vi "Demo_3 - Channel device_SetXYZRange.vi"() -> ()   [LabVIEW 2011]
uses:
  <instrlib>/Thorlabs_MDT69xB/Thorlabs_MDT69xB.lvlib
panel:
  out "Get Z voltage(V)":dbl
  out "Get Y voltage(V)":dbl
  out "Get X voltage(V)":dbl
  in  "Set Z Voltage(V)":dbl
  in  "Set Y Voltage(V)":dbl
  in  "Set x Voltage(V)":dbl
  out "Get z max voltage(V)":dbl
  out "Get z min voltage(V)":dbl
  out "Get y max voltage(V)":dbl
  out "Get y min voltage(V)":dbl
  in  "Set z max Voltage(V)":dbl=75.0
  in  "Set z min Voltage(V)":dbl
  in  "Set y max Voltage(V)":dbl=75.0
  in  "Set y min Voltage(V)":dbl
  out "Get x max voltage(V)":dbl
  out "Get x min voltage(V)":dbl
  in  "Set x max Voltage(V)":dbl=75.0
  in  "Set x min Voltage(V)":dbl
  out "v limit(V)":dbl
  out "?":string
  # "Device Info"
  # "Set Params"
  # "Get Params"
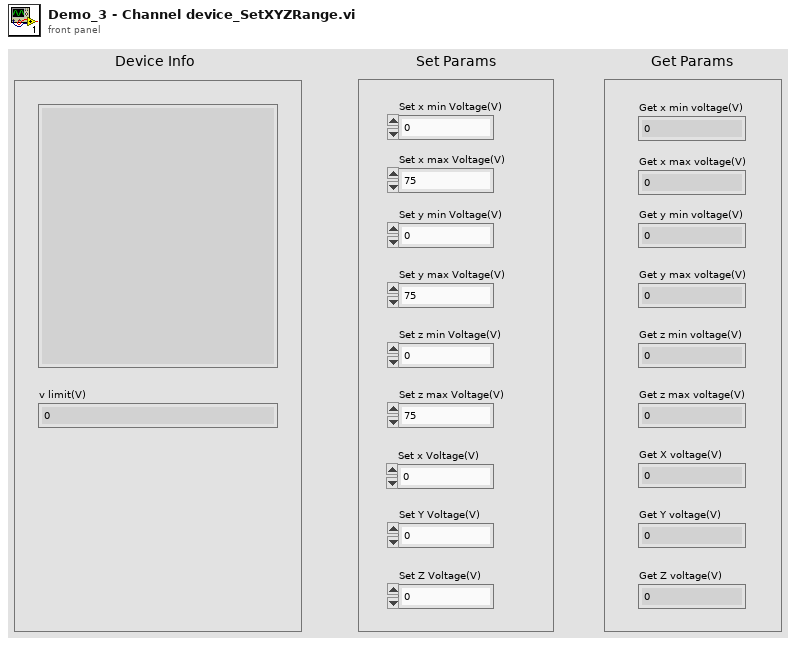
[diagram p1: front panel]
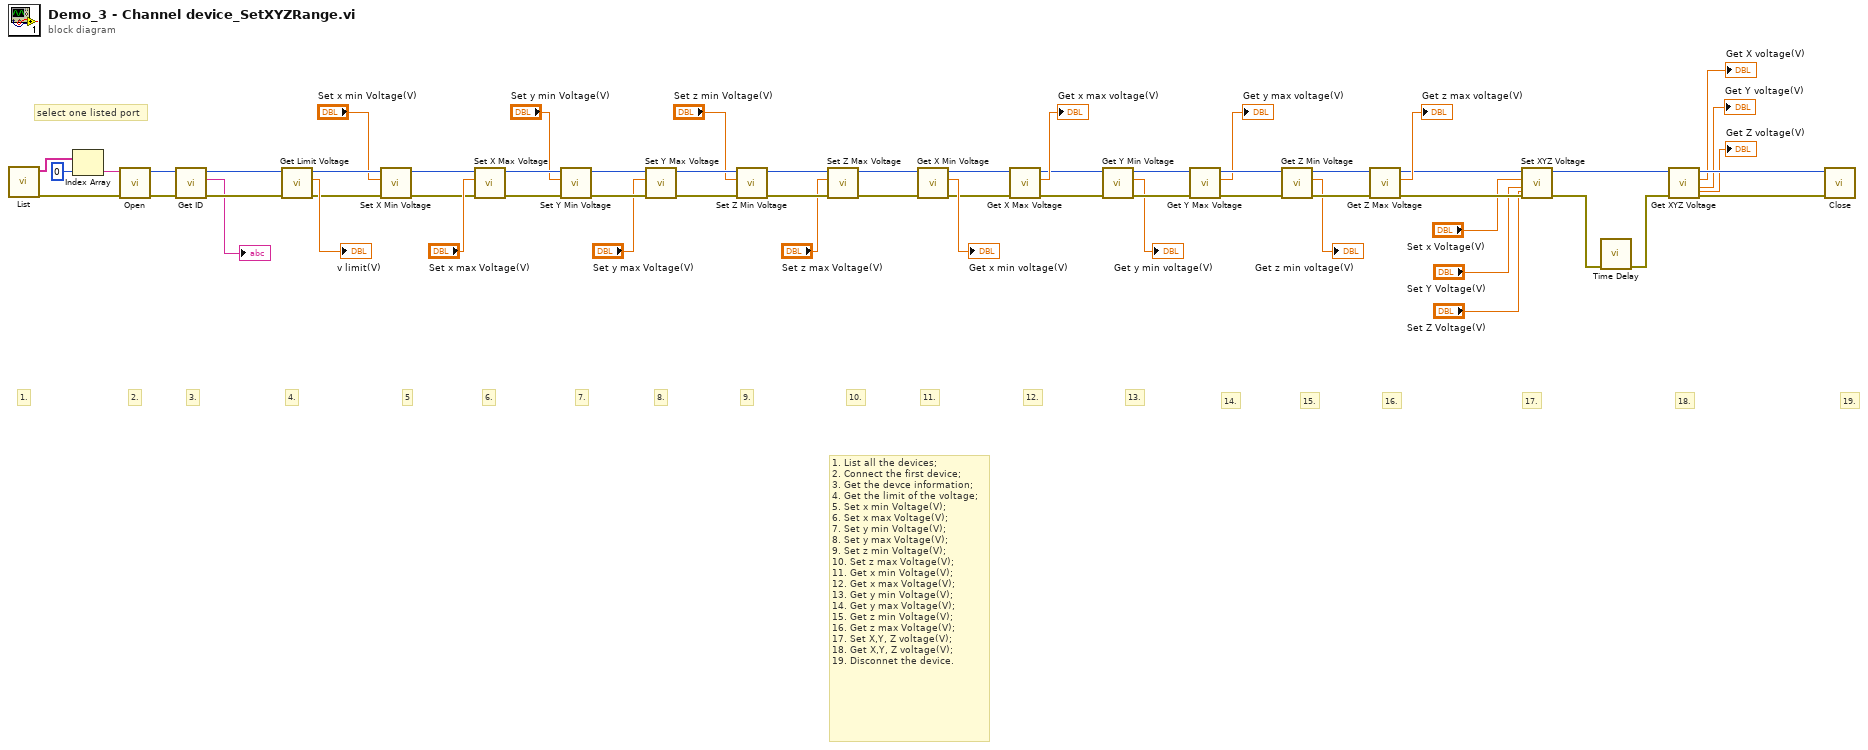
[diagram p0: block diagram]
diagram:
  # "19."
  # "18."
  # "17."
  # "16."
  # "15."
  # "14."
  # "13."
  # "12."
  # "10."
  # "9."
  # "8."
  # "7."
  # "6."
  # "5"
  # "1. List all the devices;\n2. Connect the first device;\n3. Get the devce information;\n4. Get the limit of the voltage;\n5. Set x min Voltage(V);\n6. Set x max Voltage(V);\n7. Set y min Voltage(V);\n8. Set y max Voltage(V);\n9. Set z min Voltage(V);\n10. Set z max Voltage(V);\n11. Get x min Voltage(V);\n12. Get x max Voltage(V);\n13. Get y min Voltage(V);\n14. Get y max Voltage(V);\n15. Get z min Voltage(V);\n16. Get z max Voltage(V);\n17. Set X,Y, Z voltage(V);\n18. Get X,Y, Z voltage(V);\n19. Disconnet the device."
  # "11."
  # "4."
  # "3."
  # "2."
  # "1."
  # "select one listed port"
  n1 = call <instrlib>:"List.vi"() -> ("error out"=w56:errorcluster, "COM ports"=w59:string[])  [unwired: 10 in]
  n2 = Index Array(array=w59, index=0) -> (element=w57:string)
  n3 = call <instrlib>:"Open.vi"("error in (no error)"=w56, "Serial Port"=w57) -> ("error out"=w55:errorcluster, "hDevice"=w54:i32)  [unwired: 7 in, 1 out]
  n4 = call <instrlib>:"Get ID.vi"("error in (no error)"=w55, "hdl in"=w54) -> ("error out"=w51:errorcluster, "ID"=→"?":string, "hdl out"=w53:i32)  [unwired: 7 in]
  n5 = call <instrlib>:"Get Limit Voltage.vi"("error in (no error)"=w51, "hdl in"=w53) -> ("error out"=w47:errorcluster, "v limit"=→"v limit(V)":dbl, "hdl out"=w52:i32)  [unwired: 7 in]
  n6 = call <instrlib>:"Set X Min Voltage.vi"("error in (no error)"=w47, "Set x min Voltage(V)"="Set x min Voltage(V)", "hdl in"=w52) -> ("error out"=w42:errorcluster, "hdl"=w43:i32)  [unwired: 7 in]
  n7 = call <instrlib>:"Set X Max Voltage.vi"("error in (no error)"=w42, "Set x max Voltage(V)"="Set x max Voltage(V)", "hdl in"=w43) -> ("error out"=w40:errorcluster, "hdl"=w41:i32)  [unwired: 7 in]
  n8 = call <instrlib>:"Set Y Min Voltage.vi"("error in (no error)"=w40, "Set y min Set y min Voltage(V)"="Set y min Voltage(V)", "hdl in"=w41) -> ("error out"=w38:errorcluster, "hdl"=w39:i32)  [unwired: 7 in]
  n9 = call <instrlib>:"Set Y Max Voltage.vi"("error in (no error)"=w38, "Set y max Voltage(V)"="Set y max Voltage(V)", "hdl in"=w39) -> ("error out"=w36:errorcluster, "hdl"=w37:i32)  [unwired: 7 in]
  n10 = call <instrlib>:"Set Z Min Voltage.vi"("error in (no error)"=w36, "Set z min Voltage(V)"="Set z min Voltage(V)", "hdl in"=w37) -> ("error out"=w34:errorcluster, "hdl"=w35:i32)  [unwired: 7 in]
  n11 = call <instrlib>:"Set Z Max Voltage.vi"("error in (no error)"=w34, "Set z max Voltage(V)"="Set z max Voltage(V)", "hdl in"=w35) -> ("error out"=w32:errorcluster, "hdl"=w33:i32)  [unwired: 7 in]
  n12 = call <instrlib>:"Get X Min Voltage.vi"("error in (no error)"=w32, "hdl in"=w33) -> ("error out"=w30:errorcluster, "Get x min voltage(V)"=→"Get x min voltage(V)":dbl, "hdl"=w31:i32)  [unwired: 7 in]
  n13 = call <instrlib>:"Get X Max Voltage.vi"("error in (no error)"=w30, "hdl in"=w31) -> ("error out"=w28:errorcluster, "Get x max voltage(V)"=→"Get x max voltage(V)":dbl, "hdl"=w29:i32)  [unwired: 7 in]
  n14 = call <instrlib>:"Get Y Min Voltage.vi"("error in (no error)"=w28, "hdl in"=w29) -> ("error out"=w26:errorcluster, "Get y min voltage(V)"=→"Get y min voltage(V)":dbl, "hdl"=w27:i32)  [unwired: 7 in]
  n15 = call <instrlib>:"Get Y Max Voltage.vi"("error in (no error)"=w26, "hdl in"=w27) -> ("error out"=w24:errorcluster, "Get y max voltage(V)"=→"Get y max voltage(V)":dbl, "hdl"=w25:i32)  [unwired: 7 in]
  n16 = call <instrlib>:"Get Z Min Voltage.vi"("error in (no error)"=w24, "hdl in"=w25) -> ("error out"=w22:errorcluster, "Get z min voltage(V)"=→"Get z min voltage(V)":dbl, "hdl"=w23:i32)  [unwired: 7 in]
  n17 = call <instrlib>:"Get Z Max Voltage.vi"("error in (no error)"=w22, "hdl in"=w23) -> ("error out"=w12:errorcluster, "Get z max voltage(V)"=→"Get z max voltage(V)":dbl, "hdl"=w13:i32)  [unwired: 7 in]
  n18 = call <instrlib>:"Set XYZ Voltage.vi"("Set Z Voltage(V)"="Set Z Voltage(V)", "error in (no error)"=w12, "Set Y Voltage(V)"="Set Y Voltage(V)", "Set x Voltage(V)"="Set x Voltage(V)", "hdl in"=w13) -> ("error out"=w8:errorcluster, "hdl"=w11:i32)  [unwired: 5 in]
  n19 = call "Time Delay"("error in (no error)"=w8) -> ("error out"=w7:errorcluster)  [unwired: 10 in]
  n20 = call <instrlib>:"Get XYZ Voltage.vi"("error in (no error)"=w7, "hdl in"=w11) -> ("error out"=w9:errorcluster, "Get Y voltage(V)"=→"Get Y voltage(V)":dbl, "Get X voltage(V)"=→"Get X voltage(V)":dbl, "hdl"=w10:i32, "Get Z voltage(V)"=→"Get Z voltage(V)":dbl)  [unwired: 5 in]
  n21 = call <instrlib>:"Close.vi"("error in (no error)"=w9, "hDevice"=w10) -> ()  [unwired: 9 in, 1 out]
